vi "TDT-Ramp Down.vi"(0 "RPcoX in":refnum<k7>, 7 "Ramp":bool=TRUE, 9 "Timeout (ms)":dbl=2000.0, 11 "error in (no error)":errorcluster) -> (4 "RPcoX out":refnum<k7>, 15 "error out":errorcluster)   [LabVIEW 2020]
uses:
  Utility VIs/Controls/Utilities-Wait.vi/89bc9713-8f2c-40bd-a11f-1c800a437687.vi
  <vilib>/Utility/High Resolution Polling Wait.vi
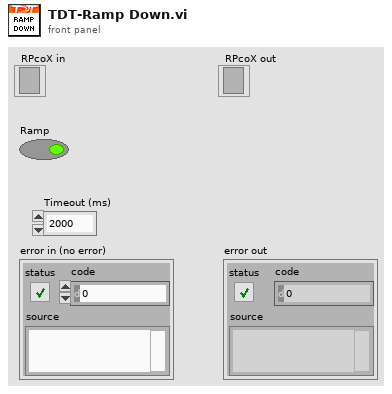
[diagram p1: front panel]
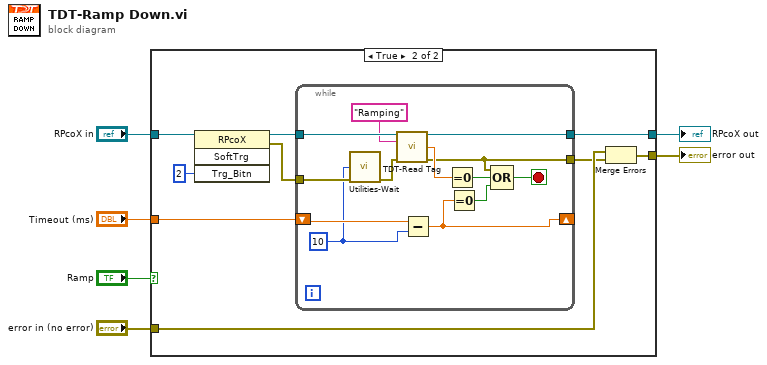
[diagram p0: block diagram]
diagram:
  n1 = case shown="True" "Ramp" {
    tunnel: "error in (no error)" -> [w7 w10]
    tunnel: "RPcoX in" -> [w8 w17]
    tunnel: [w8 w13] -> w5
    tunnel: [w7 w11] -> w6
    tunnel: "Timeout (ms)" -> [_ w12]
    frame False {
    }
    frame True {
      n2 = invoke class="RPcoX" method="SoftTrg"(reference=w17, "Trg_Bitn"=2) -> (reference out=w15:refnum<k7>, error out=w14:errorcluster)  [unwired: 2 in, 2 out]
      n3 = while {
        tunnel: w15 -> [w30]
        tunnel: w14 -> [w20]
        tunnel: [w29] -> w13
        tunnel: [w22] -> w9
        shift-right: [w21] -> _
        shift-left: w12 -> [w26]
        stop <- w23 stop-if-true
        w18 = u32 10 ("milliseconds to wait")
        n4 = call "Utilities-Wait.vi"("milliseconds to wait"=w18, "error in (no error)"=w20) -> ("error out"=w19:errorcluster)  [unwired: 13 in]
        n5 = call "TDT-Read Tag.vi"("RPcox"=w30, "Name"="Ramping", "error in"=w19) -> ("RPcox Out"=w29:refnum<k7>, "GetTagVal"=w27:sgl, "error out"=w22:errorcluster)  [unwired: 10 in]
        n6 = Subtract(x=w26, y=w18) -> (x-y=w21:dbl)
        n7 = Equal To 0?(x=w27) -> (x = 0?=w25:bool)
        n8 = Equal To 0?(x=w21) -> (x = 0?=w24:bool)
        n9 = Compound Arithmetic op=OR(w22, w25, w24) -> (w23:bool)
      }
      n10 = Merge Errors(w10, w9) -> (w11:errorcluster)
    }
  }
  "error out" <- w6
  "RPcoX out" <- w5
